vi "Read Array Key (U32).vi"(7 "Section Name":string, 8 "error in (no error)":errorcluster, 9 "Default":u32, 10 "Key Name":string, 11 "Config in":refnum<class "LabVIEW-Config.lvclass">) -> (0 "error out":errorcluster, 1 "Value":u32[](array[numeric]), 2 "Key Found?":bool, 3 "Config out":refnum<class "LabVIEW-Config.lvclass">)   [LabVIEW 2017, in "LabVIEW-Config.lvlib" / "LabVIEW-Config.lvclass"]
uses:
  LabVIEW-Config.lvclass
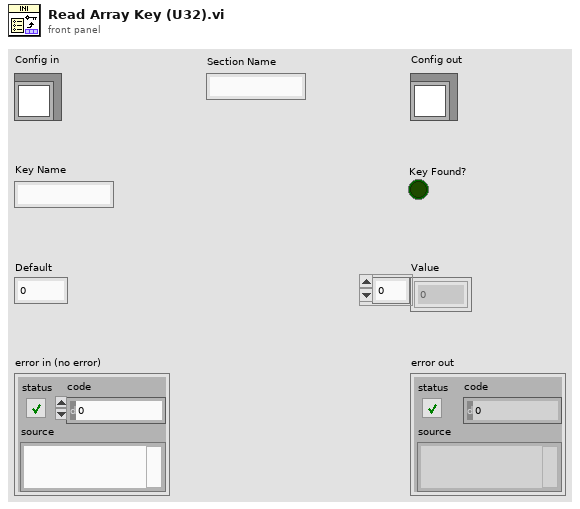
[diagram p1: front panel]
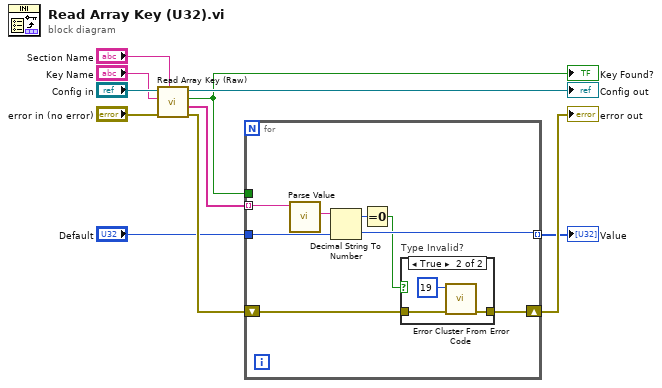
[diagram p0: block diagram]
diagram:
  n1 = call "Read Array Key (Raw).vi"("Section Name"="Section Name", "error in (no error)"="error in (no error)", "Key Name"="Key Name", "Config in"="Config in") -> ("error out"=w4:errorcluster, "Content"=w6:string[], "Key Found?"=w3:bool, "Config out"=→"Config out":refnum<class "LabVIEW-Config.lvclass">)  [unwired: 4 in]
  "Key Found?" <- w3
  n2 = for {
    tunnel: w6 -> [w19] mode=indexing
    tunnel: w3 -> [_]
    shift-right: [w18] -> w5
    shift-left: w4 -> [w17]
    tunnel: "Default" -> [w16]
    tunnel: [w15] -> w1 mode=indexing
    n3 = call "Parse Value.vi"("Value"=w19) -> ("Value (Comment Removed)"=w13:string)  [unwired: 9 in, 1 out]
    n4 = Decimal String To Number(string=w13, default (0L)=w16) -> (offset past number=w14:i32, number=w15:u32)  [unwired: 1 out]
    n5 = Equal To 0?(x=w14) -> (x = 0?=w12:bool)
    n6 = case "Type Invalid?" shown="True" w12 {
      tunnel: w17 -> [w20 w22]
      tunnel: [w20 w21] -> w18
      frame False {
      }
      frame True {
        n7 = call <vilib>:"Error Cluster From Error Code.vi"("error in (no error)"=w22, "error code (0)"=19 ("Type invalid")) -> ("error out"=w21:errorcluster)  [unwired: 7 in]
      }
    }
  }
  "error out" <- w5
  "Value" <- w1
